vi "Get Scalar Bitfile Objects.vi"(8 "error in":errorcluster, 11 "item ref in":T1 format="%.0x") -> (0 "error out":errorcluster, 1 "bitfile object names":string[](array[string]), 2 "section children refs":T1[](array[typedef]) format="%.0x", 3 "item ref out":T1 format="%.0x")   [LabVIEW 2020, in "FPGA Addon System Explorer.lvlib"]
uses:
  FPGA Addon System Explorer.lvlib
  <vilib>/NI VeriStand/Custom Device API/Custom Device Item Ref.ctl
  Addon Shared/SubVIs/Constants.vi
  <vilib>/NI VeriStand/Custom Device API/Get Item Property (String).vi
  <vilib>/NI VeriStand/Custom Device API/Custom Device API.lvlib
  Addon Shared/FPGA Addon Shared.lvlib
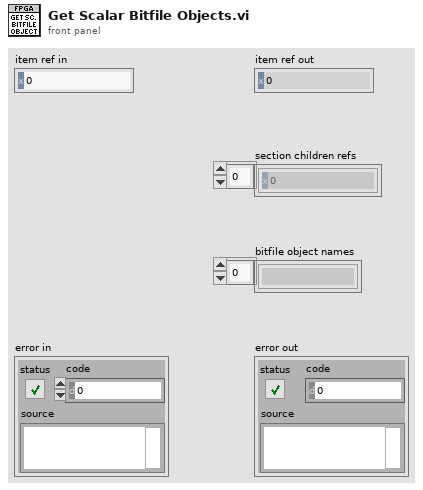
[diagram p1: front panel]
types:
  T1 = typedef "Custom Device API.lvlib/Custom Device Item Ref.ctl" = u64
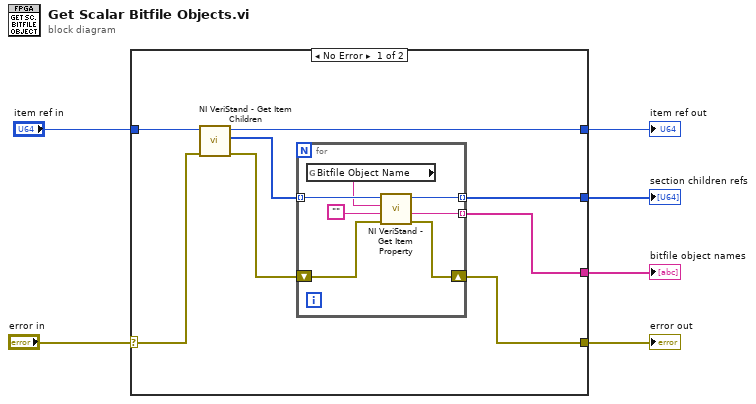
[diagram p0: block diagram]
diagram:
  n1 = case shown="No Error" "error in" {
    selector: "error in" -> [w7 w23]
    tunnel: [w14 _] -> w6
    tunnel: [w13 w23] -> w5
    tunnel: [w10 w22] -> w4
    tunnel: [w9 _] -> w3
    tunnel: "item ref in" -> [w8 w22]
    frame No Error {
      n2 = call <vilib>:"NI VeriStand - Get Item Children.vi"("error in (no error)"=w7, "Item Ref in"=w8) -> ("error out"=w12:errorcluster, "Child Refs"=w11:T1[], "Item Ref out"=w10:T1)  [unwired: 6 in, 1 out]
      n3 = for {
        shift-right: [w15] -> w13
        shift-left: w12 -> [w21]
        tunnel: w11 -> [w20] mode=indexing
        tunnel: [w19] -> w9 mode=indexing
        tunnel: [w16] -> w14 mode=indexing
        n4 = global read "Constants.vi" "Bitfile Object Name"() -> (w17:string)
        n5 = call-poly <vilib>:"NI VeriStand - Get Item Property.vi"("error in (no error)"=w21, "Default Value"="", "Property Name"=w17, "Item Ref in"=w20) -> ("error out"=w15:errorcluster, "Value"=w19:string, "Item Ref out"=w16:T1)  [unwired: 4 in, 1 out]
      }
    }
    frame Error {
    }
  }
  "section children refs" <- w6
  "error out" <- w5
  "item ref out" <- w4
  "bitfile object names" <- w3
